vi "Func1.vi"(8 "error in (no error)":errorcluster, 11 "Base in":refnum<class "Base.lvclass">) -> (0 "error out":errorcluster, 3 "Base out":refnum<class "Base.lvclass">)   [LabVIEW 2014, in "Framework.lvlib" / "Base.lvclass"]
uses:
  Base.lvclass
panel:
  in  "message":string
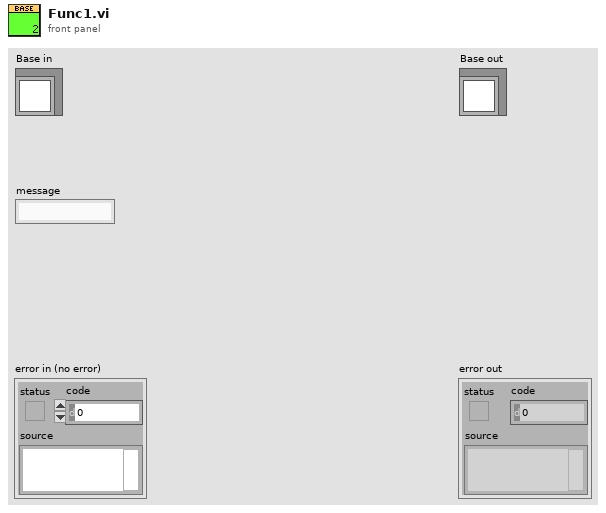
[diagram p1: front panel]
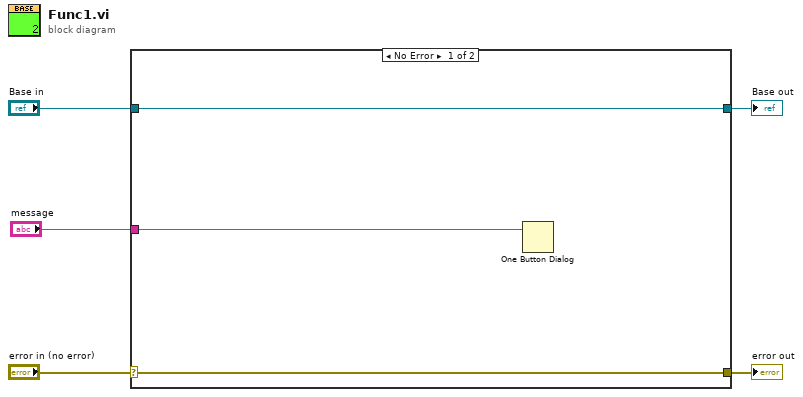
[diagram p0: block diagram]
diagram:
  n1 = case shown="No Error" "error in (no error)" {
    selector: "error in (no error)" -> [w7 w10]
    tunnel: [w7 w10] -> w4
    tunnel: [w8 w9] -> w2
    tunnel: "Base in" -> [w8 w9]
    tunnel: "message" -> [w6 _]
    frame No Error {
      n2 = One Button Dialog(message=w6) -> ()  [unwired: 1 in, 1 out]
    }
    frame Error {
    }
  }
  "error out" <- w4
  "Base out" <- w2
